vi "Read Config Unitest.vi"(8 "error in (no error)":errorcluster, 11 "main ref":T1) -> (0 "error out":errorcluster)   [LabVIEW 2025]
uses:
  controls/LAB-IQ UI Data.ctl
  Traction Loop/Traction Receipe Enum.ctl
  Config file  FGV Unitest enum.ctl
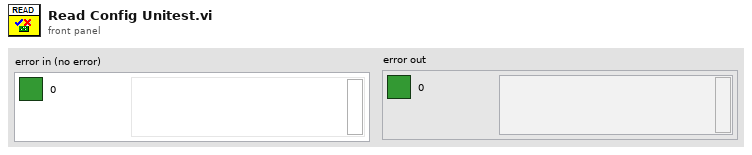
[diagram p1: front panel]
types:
  T1 = typedef "LAB-IQ UI Data.ctl" = cluster{"Main Home Screen":cluster{"GUI":refnum<vi>, "Platform Settings":refnum<vi>, "Configure":refnum<vi>, "Home":refnum<vi>, "EXIT":refnum<vi>, "service 2":refnum<vi>, "MainPage":refnum<vi>, "Analysis":refnum<vi>}, "Platform Settings":cluster{"mm/s  Surge":refnum<vi>, "Update Surge Speed":refnum<vi>, "Drive Error":refnum<vi>, "Disable Axis Jog Soft Limits":refnum<vi>, "mm/s  Sway":refnum<vi>, "Sway and Surge COM Status":refnum<vi>, "Heave COM Status":refnum<vi>, "Enable Platform":refnum<vi>, "Surge Forward Main":refnum<vi>, "Sway Right Main":refnum<vi>, "Sway Left Main":refnum<vi>, "Heave Down Main":refnum<vi>, "Heave Up main":refnum<vi>, "Update Sway Speed":refnum<vi>, "Update Heave Speed":refnum<vi>, "mm/s Heave":refnum<vi>, "mm/sec":refnum<vi>, "mm":refnum<vi>, "Surge Backward Main":refnum<vi>}, "Analysis Screen":cluster{"Analysis Home":refnum<vi>, "Surface Analysis":refnum<vi>, "Imaging":refnum<vi>, "Image Analysis":refnum<vi>, "Post Analysis":refnum<vi>}, "Config Screen":cluster{"Select Load Head":refnum<vi>, "Notes :":refnum<vi>, "FILE":refnum<vi>, "Sample ID :":refnum<vi>, "Operator ID :":refnum<vi>, "Operator Name :":refnum<vi>, "Auto":refnum<vi>}, "Motion Module":cluster{"zNL":refnum<vi>, "NL disp":refnum<vi>, "Rotary Tab":refnum<vi>, "Motion Direction:  3":refnum<vi>, "E.Velocity 2":refnum<vi>, "e.v/ssr 2":refnum<vi>, "Enter Fixed E.Velocity 2":refnum<vi>, "Enter Final SRR 2":refnum<vi>, "Enter initial SRR 2":refnum<vi>, "Enter Fixed SRR 2":refnum<vi>, "Enter the Final E.Velocity (m/s) 2":refnum<vi>, "Enter initial E.Velocity (m/s) 2":refnum<vi>, "Final Speed (RPM) 3":refnum<vi>, "Initial Speed (RPM) 2":refnum<vi>, "Enter the Final Velocity (m/s) 3":refnum<vi>, "Enter initial Velocity (m/s)  3":refnum<vi>, "Ramp Up 2":refnum<vi>, "TEST SELECTION":refnum<vi>, "SPEED SELECTION : ":refnum<vi>, "Angular Oscillation Set":refnum<vi>, "Traction":refnum<vi>, "Step Speed":refnum<vi>, "StepTable For Load-Speed":refnum<vi>, "StepTable For Speed":refnum<vi>, "Surge Forward MM":refnum<vi>, "Surge Backward MM":refnum<vi>, "M3 Image":refnum<vi>, "String 39":refnum<vi>, "Sway Left MM":refnum<vi>, "Sway Right MM":refnum<vi>, "Disable Axis Jog Soft Limits":refnum<vi>, "mm":refnum<vi>, "Heave Down MM":refnum<vi>, "Heave Up MM":refnum<vi>, "Wear Track Diameter (mm)":refnum<vi>, "Set WTD":refnum<vi>, "HomeScratch":refnum<vi>, "HomeRot":refnum<vi>, "PlaceModule":refnum<vi>, "Enter the Angle (Deg)":refnum<vi>, "Enter the Frequency (Hz)":refnum<vi>, "Motion Mode:":refnum<vi>, "LR Sway":refnum<vi>, "Rot Hor":refnum<vi>, "Scratch":refnum<vi>, "LR Cam":refnum<vi>, "MMBack":refnum<vi>, "MMNext":refnum<vi>, "Rot Ver":refnum<vi>, "Rotary Module Selection":refnum<vi>, "calculate rotary":refnum<vi>, "SPEED SELECTION : rotary":refnum<vi>, "Import 2":refnum<vi>, "Save 2":refnum<vi>, "File Path :  2":refnum<vi>, "String 45":refnum<vi>, "StepTable For Speed 3":refnum<vi>, "Enter the Speed(mm/sec)":refnum<vi>, "Enter the Speed(RPM)":refnum<vi>, "Enter Scratch Speed (mm/s):":refnum<vi>, "SwaySpeed Set":refnum<vi>, "Scartch Offset":refnum<vi>, "Motion type:":refnum<vi>, "HomeScratch 2":refnum<vi>, "Enter Scratch length (mm):":refnum<vi>, "Wear Track Diameter":refnum<vi>, "Rotary Speed Exced":refnum<vi>, "Scratch Mode":refnum<vi>, "No of Scratch":refnum<vi>}, "Environmental control":cluster{"Humidity  Status  3":refnum<vi>, "Low Temp  Status  2":refnum<vi>, "TK4 status 2":refnum<vi>, "Stage Temperature":refnum<vi>, "Sample Temperature":refnum<vi>, "Humidity (Amb)":refnum<vi>, "Clear List":refnum<vi>, "Add to list":refnum<vi>, "Wear":refnum<vi>, "Vibration":refnum<vi>, "Humidity (Chamber)":refnum<vi>, "Temperature (Chamber)":refnum<vi>, "ECR ":refnum<vi>, "Temperature (Amb)":refnum<vi>, "Microphone":refnum<vi>, "Acoustic Emission 3":refnum<vi>, "SNext":refnum<vi>, "APBack":refnum<vi>, "Enter the Temperature (°C):":refnum<vi>, "Enter the Stage \nTemperature (°C):":refnum<vi>, "Enter the Humidity (%Rh):":refnum<vi>, "Low Temp":refnum<vi>, "High Temp":refnum<vi>, "Humidity":refnum<vi>, "Sensors Picked":refnum<vi>}, "About Screen":cluster{"Password":refnum<vi>, "Home Service":refnum<vi>, "Advanced Setting":refnum<vi>, "About Tab":refnum<vi>, "ECR Port:":refnum<vi>, "Ramp Port:":refnum<vi>, "Installation/Replacement completed":refnum<vi>, "Loahead":refnum<vi>, "Heave and Surge COM Port:":refnum<vi>, "Sway COM Port:":refnum<vi>, "Temp Modbus:":refnum<vi>, "Humidity Port:":refnum<vi>, "Edit Gain Constants":refnum<vi>, "Save Gain Constants":refnum<vi>}, "Main Screen":cluster{"Main Screen Tab":refnum<vi>, "Angle and Frequency":refnum<vi>, "Stroke (mm)":refnum<vi>, "Angle (Deg)":refnum<vi>, "Main Speed Tab":refnum<vi>, "MTM MOTOR DISPLAY":refnum<vi>, "Disc Speed (m/sec)":refnum<vi>, "Ball Speed (m/sec)":refnum<vi>, "Disc Speed (RPM)":refnum<vi>, "Ball Speed (RPM)":refnum<vi>, "SPEED TAB":refnum<vi>, "Speed (m/sec)":refnum<vi>, "Set Speed (m/sec)":refnum<vi>, "Speed (RPM)":refnum<vi>, "Set Speed":refnum<vi>, "Time Tab":refnum<vi>, "Time ( HH:MM:SS ) 2":refnum<vi>, "Test Duration":refnum<vi>, "Test Duration 4":refnum<vi>, "TEST CYCLE":refnum<vi>, "TOTAL CYCLES":refnum<vi>, "Set Load (N)":refnum<vi>, "Temp Tabs":refnum<vi>, "Heater":refnum<vi>, "TK4 status":refnum<vi>, "ChamberTemp":refnum<vi>, "SetTmp":refnum<vi>, "Controller  Status":refnum<vi>, "ChamberTemp 2":refnum<vi>, "SetTmp 2":refnum<vi>, "Controller  Status 2":refnum<vi>, "ChamberTemp 3":refnum<vi>, "SetTmp 3":refnum<vi>, "Cooling":refnum<vi>, "Load Communication":refnum<vi>, "Ambient \nTemperature":refnum<vi>, "HumCOMStatus":refnum<vi>, "Ambient\n Humidity":refnum<vi>, "Freq (Hz)":refnum<vi>, "Load En":refnum<vi>, "NLt":refnum<vi>, "zNL 2":refnum<vi>, "Humidity On":refnum<vi>, "humidity disp":refnum<vi>, "Set Humidity":refnum<vi>, "NL disp 2":refnum<vi>, "Humidity On 2":refnum<vi>, "humidity disp 2":refnum<vi>, "Set Humidity 2":refnum<vi>, "NL disp 3":refnum<vi>, "AppLoadSeq scratch":refnum<vi>, "Stop Scratch":refnum<vi>, "ClrLog":refnum<vi>, "Trip Log":refnum<vi>, "STOP":refnum<vi>, "Start Test":refnum<vi>, "Test status":refnum<vi>, "AR Led":refnum<vi>, "Data":refnum<vi>, "Health":refnum<vi>, "Sway COM Status":refnum<vi>, "Heave COM Status":refnum<vi>, "Grp Tab":refnum<vi>, "Sub Graph":refnum<vi>, "SD (mm)":refnum<vi>, "Siliding distance Reset Graph":refnum<vi>, "SDGp":refnum<vi>, "Humidity Reset Graph":refnum<vi>, "HumrGp":refnum<vi>, "Acoustic Emission (mV)":refnum<vi>, "Aqucostic Reset Graph":refnum<vi>, "gACQUOS":refnum<vi>, "ECR RESET":refnum<vi>, "ECR":refnum<vi>, "Temperature Reset":refnum<vi>, "Acoustic Emission (mV) 2":refnum<vi>, "Aqucostic Reset Graph 2":refnum<vi>, "gACQUOS 2":refnum<vi>, "ECR RESET 2":refnum<vi>, "ECR 2":refnum<vi>, "Temperature Reset 2":refnum<vi>, "Temperature (deg c)":refnum<vi>, "Speed Reset Graph":refnum<vi>, "Speed Tab":refnum<vi>, "MTM DISC  SPEED":refnum<vi>, "MTM BALL SPEED":refnum<vi>, "speed mm/sec":refnum<vi>, "Hymidity":refnum<vi>, "Humidity Disable trip":refnum<vi>, "CoF Trip  2":refnum<vi>, "Depth Trip":refnum<vi>, "Weart Deapth":refnum<vi>, "Depth Reset Graph":refnum<vi>, "Weart":refnum<vi>, "Depthz":refnum<vi>, "Depth (µm)":refnum<vi>, "WearGp":refnum<vi>, "NL Trip 2":refnum<vi>, "Load pid":refnum<vi>, "Load Disable Trip":refnum<vi>, "Load Reset Graph":refnum<vi>, "NL Display 4":refnum<vi>, "Main Chart 3":refnum<vi>, "BACK":refnum<vi>, "Depth Trip 2":refnum<vi>, "COF TRIP ":refnum<vi>, "Friction Force (N)":refnum<vi>, "FF Reset Graph":refnum<vi>, "FF Disable Trip":refnum<vi>, "FF TRIP":refnum<vi>, "COF Disable Trip":refnum<vi>, "COF Reset Graph":refnum<vi>, "Start Test Temp":refnum<vi>, "zFF":refnum<vi>, "Friction Force (N) Graph":refnum<vi>, "Coefficient of Friction":refnum<vi>, "Scratch Start Test":refnum<vi>, "FF Tab":refnum<vi>, "Cyclic Friction Force (N)":refnum<vi>, "CZ FF":refnum<vi>, "Cyclic Friction Force (N) Graph":refnum<vi>, "Cyclic Coefficient of Friction":refnum<vi>, "Cyclic FF TRIP":refnum<vi>, "Cyclic FF Disable Trip":refnum<vi>, "cyclic COF Disable Trip":refnum<vi>, "cyclic COF TRIP":refnum<vi>, "cyclic COF Reset Graph":refnum<vi>, "Cyclic FF Reset Graph":refnum<vi>, "Test Trip":refnum<vi>, "Multi Scratch Pass":refnum<vi>, "Scratch Start Recording":refnum<vi>}, "Loading":cluster{"Indentation":refnum<vi>, "Reference Sample":refnum<vi>, "Load Cell Communication Slide":refnum<vi>, "com 3":refnum<vi>, "com":refnum<vi>, "DecaForce COM Status":refnum<vi>, "Update":refnum<vi>, "Clear 3":refnum<vi>, "seq":refnum<vi>, "Stribeck table":refnum<vi>, "Stribeck Table  For loading":refnum<vi>, "Loading Mode":refnum<vi>, "Enter the Final Load (N)":refnum<vi>, "Enter the CoF Trip":refnum<vi>, "Enter the Friction Force Trip":refnum<vi>, "Enter the Normal load Trip":refnum<vi>, "Enter the Load  (N)":refnum<vi>, "KiloForce":refnum<vi>, "DecaForce ":refnum<vi>, "MicroForce":refnum<vi>, "LHBack":refnum<vi>, "LHNext":refnum<vi>, "Enter the Loading Rate (N/min)":refnum<vi>, "Message":refnum<vi>, "Warning 2":refnum<vi>, "SSP 0.75":refnum<vi>, "SSP 0.5":refnum<vi>, "SSP 0.3":refnum<vi>, "Warning":refnum<vi>, "gui GIF":refnum<vi>, "Communication is established":refnum<vi>, "AppLoad 4":refnum<vi>, "Multipoint":refnum<vi>, "Load Selection":refnum<vi>}, "PID":cluster{"Ramp MulFac":refnum<vi>, "pulses LoadDiffRamp(2..10)":refnum<vi>, "PulseControlRamp(diff<=3N)":refnum<vi>, "SetLoadDeadband(%) Load(0-10N)":refnum<vi>, "PID gains out delay (microForce)":refnum<vi>, "Ramp":refnum<vi>, "Gain 2":refnum<vi>, "pulses LoadDiff(2..10)":refnum<vi>, "pulses LoadDiff(11..50)":refnum<vi>, "PulseControl(diff<=3N)":refnum<vi>, "SetLoadDeadband(%)  2":refnum<vi>, "Dummy Run":refnum<vi>, "Vertical load (N)":refnum<vi>, "AutoTune":refnum<vi>, "Offset 3 ":refnum<vi>, "apply load":refnum<vi>, "Offset  3":refnum<vi>, "apply load 2":refnum<vi>, "Enter ByPass Load":refnum<vi>, "reinit 3":refnum<vi>, "output range delay":refnum<vi>, "PID gains out delay":refnum<vi>, "Bypass Load":refnum<vi>, "pulsesSent":refnum<vi>, "pulses ":refnum<vi>, "actpid":refnum<vi>, "gFF Rot":refnum<vi>, "pulses LoadDiff(21..1000)":refnum<vi>, "Delay":refnum<vi>, "deadband":refnum<vi>}, "Config Parameters":cluster{"Tab Control 3":refnum<vi>, "Tab Control 19":refnum<vi>, "SAMPLES":refnum<vi>, "Re-initilaize":refnum<vi>, "Filter ON/OFF":refnum<vi>, "TracHomeSurgeOffsetCounts 10MM":refnum<vi>, "TracHomeSwayOffsetCounts 10MM":refnum<vi>, "Acoustic Emission:":refnum<vi>, "Apply Filter (FF)":refnum<vi>, "Filter% 2":refnum<vi>, "Apply Filter (Load)":refnum<vi>, "Filter% ":refnum<vi>, "Sway distance (mm)":refnum<vi>, "Surge distance (mm)":refnum<vi>, "DataSavingLoopDelay(ms)":refnum<vi>, "SAVE 2":refnum<vi>, "Enter Distance":refnum<vi>, "Sway Counts:":refnum<vi>, "Distance (mm): 3":refnum<vi>, "Surge Counts:":refnum<vi>, "Distance (mm): 2":refnum<vi>, "Distance (mm):":refnum<vi>, "Heave Counts:":refnum<vi>, "LRMHomeSurgeOffsetCounts":refnum<vi>, "LRMHomeSwayOffsetCounts":refnum<vi>, "TracHomeSurgeOffsetCounts 20MM":refnum<vi>, "TracHomeSwayOffsetCounts 20MM":refnum<vi>, "RotHomeSwayOffsetCounts":refnum<vi>, "RotHomeSurgeOffsetCounts":refnum<vi>, "Heave distance":refnum<vi>, "Zmm":refnum<vi>, "Heave Pulses/mm":refnum<vi>, "Surge Pulses/mm":refnum<vi>, "Sway Pulses/mm":refnum<vi>, "Heave Pitch":refnum<vi>, "Surge Pitch":refnum<vi>, "Sway Pitch":refnum<vi>, "Heave PPR":refnum<vi>, "Surge PPR":refnum<vi>, "Sway PPR":refnum<vi>, "Tab Control 5":refnum<vi>, "Tab Control 14":refnum<vi>, "Tab Control 26":refnum<vi>, "AE":refnum<vi>, "Heave Loop Delay":refnum<vi>, "Heave PID Speed":refnum<vi>, "Surge Jog Speed":refnum<vi>, "Heave Jog Speed":refnum<vi>, "Sway Loop Delay":refnum<vi>, "Sway PID Speed":refnum<vi>, "Sway Jog Speed":refnum<vi>, "DEPTH TRIP VALUE":refnum<vi>, "LOAD TRIP VALUE":refnum<vi>, "DEPTH TRIP   ENABLE":refnum<vi>, "LOAD TRIP  ENABLE":refnum<vi>, "CYCLIC FF TRIP VALUE":refnum<vi>, "FF TRIP VALUE":refnum<vi>, "CYCLIC CoF TRIP VALUE":refnum<vi>, "COF TRIP VALUE":refnum<vi>, "CYCLIC COF TRIP  ENABLE":refnum<vi>, "CYCLIC FF TRIP  ENABLE":refnum<vi>, "FF TRIP  ENABLE":refnum<vi>, "COF TRIP  ENABLE":refnum<vi>, "JOG TRIP LOAD VALUE (N)":refnum<vi>, "Rotary Vertical":refnum<vi>, "Traction":refnum<vi>, "Scratch":refnum<vi>, "LRM CAM":refnum<vi>, "Sway LRM":refnum<vi>, "Rotary Horizontal":refnum<vi>}, "Loading Com Port":cluster{"ClearAll":refnum<vi>, "Mz(Nm)":refnum<vi>, "My(Nm)":refnum<vi>, "Mx(Nm)":refnum<vi>, "Save Dwell":refnum<vi>, "Acq Delay (ms)":refnum<vi>, "Burst Delay (ms)":refnum<vi>, "model":refnum<vi>, "SN":refnum<vi>, "FFx(N)":refnum<vi>, "Sensor IP":refnum<vi>, "Port":refnum<vi>, "FFy(N)":refnum<vi>, "Load(N)":refnum<vi>, "delete Handle":refnum<vi>, "Create Handle":refnum<vi>, "ft_data":refnum<vi>, "ft_range":refnum<vi>, "ft_data 2":refnum<vi>, "stop 6":refnum<vi>, "running_flag":refnum<vi>, "ft_udp_handle":refnum<vi>, "get-data-return":refnum<vi>, "get-range-return":refnum<vi>, "zero-return":refnum<vi>, "filter-return":refnum<vi>, "initial-return":refnum<vi>, "deleteHandle-result":refnum<vi>, "Load Cell Temp":refnum<vi>, "Load Cell":refnum<vi>, "ZeroAll":refnum<vi>, "FORCE (N)":refnum<vi>, "TORQUE (N-m)":refnum<vi>}, "Heave AND Surge":cluster{"SURGE POSE":refnum<vi>, "error out Read":refnum<vi>, "HEAVE POSE":refnum<vi>, "State":refnum<vi>, "Homed":refnum<vi>, "Sequence ID":refnum<vi>, "error out Write":refnum<vi>, "faultCode":refnum<vi>, "Ack ID":refnum<vi>, "SPEED":refnum<vi>, "Distance":refnum<vi>, "Mode Command":refnum<vi>, "Heave and Surge Read":refnum<vi>, "Read Heave Temp":refnum<vi>, "Spare 15":refnum<vi>, "Spare 14":refnum<vi>, "Spare 13":refnum<vi>, "Spare 12":refnum<vi>, "Spare 11":refnum<vi>, "Spare 10":refnum<vi>, "Spare 9":refnum<vi>, "Spare 8":refnum<vi>, "Spare 7":refnum<vi>, "Spare 6":refnum<vi>, "Spare 5":refnum<vi>, "Spare 4":refnum<vi>, "Spare 2":refnum<vi>, "Spare 1":refnum<vi>, "Node Id":refnum<vi>, "Spare 3":refnum<vi>, "SPARE 4":refnum<vi>, "SPARE 3":refnum<vi>, "SPARE 2":refnum<vi>, "SPARE 1":refnum<vi>, "fwMajor":refnum<vi>, "fwMinor":refnum<vi>, "Manual Write":refnum<vi>, "Heave and Surge Write":refnum<vi>, "SPARE 5":refnum<vi>, "Reserved ":refnum<vi>, "SPARE 8":refnum<vi>, "SPARE 6":refnum<vi>, "SPARE 7":refnum<vi>, "SPARE 17":refnum<vi>, "SPARE 16":refnum<vi>, "SPARE 15":refnum<vi>, "SPARE 14":refnum<vi>, "SPARE 13":refnum<vi>, "SPARE 12":refnum<vi>, "SPARE 11":refnum<vi>, "SPARE 10":refnum<vi>, "SPARE 9":refnum<vi>, "System UPTIME":refnum<vi>, "Missed Packets":refnum<vi>, "faultCode Surge Right":refnum<vi>, "faultCode Surge Left":refnum<vi>, "faultCode Heave":refnum<vi>, "UPLINK HEAVE":refnum<vi>, "DOWNLINK HEAVE":refnum<vi>}, "New PID LOGIC":cluster{"Fine Tune Zone":refnum<vi>, "PID SDelay":refnum<vi>, "Max_pos_limit":refnum<vi>, "Min_pos_limit":refnum<vi>, "i_limit":refnum<vi>, "pct_scale":refnum<vi>, "Deadband":refnum<vi>, "Kd":refnum<vi>, "Ki":refnum<vi>, "Kp":refnum<vi>, "Current Position":refnum<vi>, "Set Load":refnum<vi>, "Current Load":refnum<vi>, "Pulse delta":refnum<vi>, "Init Step":refnum<vi>, "Max Step Linit":refnum<vi>, "min_deadband_floor":refnum<vi>, "dynamic_spindle_noise_scalar":refnum<vi>, "min_finetune_floor":refnum<vi>, "filter_alpha":refnum<vi>, "PID":refnum<vi>}, "SWAY ":cluster{"fwMajor":refnum<vi>, "Homed":refnum<vi>, "Rotary POSE":refnum<vi>, "State":refnum<vi>, "SWAY POSE":refnum<vi>, "Ack ID":refnum<vi>, "faultCode":refnum<vi>, "Node Id":refnum<vi>, "fwMinor":refnum<vi>, "Spare 6":refnum<vi>, "Spare 5":refnum<vi>, "Spare 4":refnum<vi>, "Spare 3":refnum<vi>, "Spare 2":refnum<vi>, "Spare 1":refnum<vi>, "Spare 7":refnum<vi>, "SPARE  5":refnum<vi>, "error out Write  SWAY ":refnum<vi>, "error out Read SWAY ":refnum<vi>, "Manual Write SWAY ":refnum<vi>, "SWAY WRITE":refnum<vi>, "SPARE  4":refnum<vi>, "SPARE  3":refnum<vi>, "SPARE 2":refnum<vi>, "SPARE 1":refnum<vi>, "Spare 15":refnum<vi>, "Spare 14":refnum<vi>, "Spare 13":refnum<vi>, "Spare 12":refnum<vi>, "Spare 11":refnum<vi>, "Spare 9":refnum<vi>, "Spare 8":refnum<vi>, "SPEED":refnum<vi>, "Distance":refnum<vi>, "Mode Command":refnum<vi>, "Sequence ID":refnum<vi>, "SWAY READ":refnum<vi>, "Spare 10":refnum<vi>, "Read SWAY Temp":refnum<vi>, "faultCode Sway ":refnum<vi>, "Missed Packets":refnum<vi>, "System UPTIME sway":refnum<vi>, "SPARE 6":refnum<vi>, "SPARE 7":refnum<vi>, "SPARE 9":refnum<vi>, "SPARE 11":refnum<vi>, "SPARE 10":refnum<vi>, "SPARE 8":refnum<vi>, "SPARE 13":refnum<vi>, "SPARE 12":refnum<vi>, "SPARE 17":refnum<vi>, "SPARE 16":refnum<vi>, "SPARE 15":refnum<vi>, "SPARE 14":refnum<vi>, "Reserved":refnum<vi>, "faultCode Rotary":refnum<vi>, "UPLINK SWAY":refnum<vi>, "DOWNLINK SWAY":refnum<vi>}, "Analysis Screen":cluster{"Analysis Home":refnum<vi>, "Refresh 2":refnum<vi>, "MEAN 4":refnum<vi>, "SD 4":refnum<vi>, "VARIANCE 4":refnum<vi>, "MEAN  3":refnum<vi>, "SD  3":refnum<vi>, "VARIANCE  3":refnum<vi>, "MEAN 2":refnum<vi>, "SD  2":refnum<vi>, "VARIANCE 2":refnum<vi>, "MEAN":refnum<vi>, "SD":refnum<vi>, "VARIANCE":refnum<vi>, "File 4 Discription":refnum<vi>, "OPEN 4":refnum<vi>, "File Name 4":refnum<vi>, "OPEN 3":refnum<vi>, "File 3 Discription":refnum<vi>, "File Name 3":refnum<vi>, "Y-AXIS":refnum<vi>, "X-AXIS":refnum<vi>, "XY Graph":refnum<vi>, "File Name 2":refnum<vi>, "File Name 1":refnum<vi>, "OPEN 2":refnum<vi>, "OPEN 1":refnum<vi>, "File 1 Discription ":refnum<vi>, "File 2 Discription":refnum<vi>, "Export":refnum<vi>, "File Format":refnum<vi>}, "Traction":cluster{"faultCode Traction 2":refnum<vi>, "faultCode Traction 1":refnum<vi>, "Missed Packets":refnum<vi>, "System UPTIME Traction":refnum<vi>, "SPARE 17":refnum<vi>, "SPARE 16":refnum<vi>, "SPARE 15":refnum<vi>, "SPARE 14":refnum<vi>, "SPARE 13":refnum<vi>, "SPARE 12":refnum<vi>, "SPARE 11":refnum<vi>, "SPARE 10":refnum<vi>, "SPARE 9":refnum<vi>, "SPARE 8":refnum<vi>, "SPARE 7":refnum<vi>, "SPARE 6":refnum<vi>, "Reserved":refnum<vi>, "SPARE  5":refnum<vi>, "Manual Write TRACTION":refnum<vi>, "TRACTION WRITE":refnum<vi>, "SPARE  4":refnum<vi>, "SPARE  3":refnum<vi>, "SPARE 2":refnum<vi>, "SPARE 1":refnum<vi>, "Spare 7":refnum<vi>, "Spare 6":refnum<vi>, "Spare 5":refnum<vi>, "Spare 4":refnum<vi>, "Spare 2":refnum<vi>, "Spare 1":refnum<vi>, "Node Id":refnum<vi>, "Read TRACTION Temp":refnum<vi>, "fwMinor":refnum<vi>, "fwMajor":refnum<vi>, "faultCode":refnum<vi>, "TRACTION POSE":refnum<vi>, "TRACTION POSE 2":refnum<vi>, "Homed":refnum<vi>, "State":refnum<vi>, "Ack ID":refnum<vi>, "SPEED":refnum<vi>, "Distance":refnum<vi>, "Mode Command":refnum<vi>, "Sequence ID":refnum<vi>, "error out Read TRACTION":refnum<vi>, "error out Write  TRACTION":refnum<vi>, "TRACTION READ":refnum<vi>, "Spare 3":refnum<vi>, "Downlink traction":refnum<vi>, "Uplink Traction":refnum<vi>}, "Traction reciepe":cluster{"SRR Sweep Range (%) Stribeck":refnum<vi>, "Traction Receipe":refnum<vi>, "Total Execution Time":refnum<vi>, "Total Steps":refnum<vi>, "Duration / Step (s)  Stribeck":refnum<vi>, "STRIBECK Fixed SRR List (%)":refnum<vi>, "Duration / Step (s) Traction":refnum<vi>, "SRR Sweep Range (%) traction":refnum<vi>, "Rolling Speed (mm/s)":refnum<vi>, "Temperature Stages (°C)":refnum<vi>, "Ball Load (N)":refnum<vi>, "Lubricant Name":refnum<vi>, "Profile File Name":refnum<vi>, "SET entrainment Velocity":refnum<vi>, "Test Array Size":refnum<vi>, "SRR INDEX [ STRIBECK]":refnum<vi>, "Stribeck Size":refnum<vi>, "SET SRR":refnum<vi>, "ELAPSED TIMER ":refnum<vi>, "BALL SET RPM":refnum<vi>, "DISC SET RPM":refnum<vi>, "SET LOAD":refnum<vi>, "TEMPERATURE READ":refnum<vi>, "SET TEMPERATURE":refnum<vi>, "Traction Size":refnum<vi>, "DISC SPEED (rpm)":refnum<vi>, "BALL SPEED (rpm)":refnum<vi>, "BALL WEAR TRACK":refnum<vi>, "DISC WEARTRACK":refnum<vi>, "SRR INDEX [ TRACTION]":refnum<vi>, "Start Index Type":refnum<vi>, "Enum - Menu":refnum<vi>, "Ball (mm/sec)":refnum<vi>, "Disc (mm/sec)":refnum<vi>}, "Traction Control":cluster{"HomeTraction":refnum<vi>, "Demo Mode Display":refnum<vi>, "Traction Message":refnum<vi>, "Traction Step Update Details":refnum<vi>, "Main Tab sequence for selection":refnum<vi>, "Ramp Tab":refnum<vi>, "e.v/ssr":refnum<vi>, "Enter Fixed E.Velocity":refnum<vi>, "Enter Final SRR":refnum<vi>, "Enter initial SRR":refnum<vi>, "Enter Fixed SRR":refnum<vi>, "Enter the Final E.Velocity (m/s)":refnum<vi>, "Enter initial E.Velocity (m/s)":refnum<vi>, "Ball WTD":refnum<vi>, "E.Velocity":refnum<vi>, "Enter the Final Velocity (m/s)":refnum<vi>, "Enter initial Velocity (m/s)":refnum<vi>, "Ramp Up   Disc":refnum<vi>, "Initial DiscSpeed (RPM)":refnum<vi>, "Final Speed (RPM) Ball":refnum<vi>, "Final Speed (RPM)":refnum<vi>, "Initial Speed (RPM) Ball":refnum<vi>, "Enter the Final Velocity (m/s) Ball":refnum<vi>, "Enter initial Velocity (m/s) Ball":refnum<vi>, "Ramp Up":refnum<vi>, "ExceedBallSpeed step":refnum<vi>, "ExceedDiscSpeed":refnum<vi>, "BallSpeed Exceed Indication":refnum<vi>, "Apply":refnum<vi>, "SPEED SELECTION : MTM":refnum<vi>, "SPEED SELECTION : MTM 2":refnum<vi>, "TEST SELECTION (MTM)":refnum<vi>, "MTM Test Selection":refnum<vi>, "File Path Tab":refnum<vi>, "File Path String":refnum<vi>, "Save":refnum<vi>, "Save  2":refnum<vi>, "Import ":refnum<vi>, "File Path :":refnum<vi>, "Step Sequence Indication Tab":refnum<vi>, "Step Sequence Indication":refnum<vi>, "Calculate Step":refnum<vi>, "StepTable":refnum<vi>, "ExceedDiscSpeed  Cinstant Speed":refnum<vi>, "ExceedBallSpeed Constant":refnum<vi>, "TEST SELECTION (MTM) 2":refnum<vi>, "SPEED SELECTION : MTM 3":refnum<vi>, "MTM Test Selection 2":refnum<vi>, "Enter the Speed (m/sec): ":refnum<vi>, "Enter the Speed (m/sec):  2":refnum<vi>, "Enter the Speed (RPM):":refnum<vi>, "Lower Spped ":refnum<vi>, "Upper":refnum<vi>, "Enter the Speed (RPM):Ball":refnum<vi>, "Disc Motion Direction: ":refnum<vi>, "Ball Motion Direction :":refnum<vi>, "Motion Mode: ":refnum<vi>, "Wear Track Diameter (mm) ":refnum<vi>, "Disc Speed Indicator":refnum<vi>, "ExceedBallSpeed":refnum<vi>}, "Acquostic":cluster{"Last Config Rejected ":refnum<vi>, "rx command count":refnum<vi>, "Current Filter Id":refnum<vi>, "Isolated Gain":refnum<vi>, "DAQ Status":refnum<vi>, "error out":refnum<vi>, "error in (no error)":refnum<vi>, "Uplink Packet":refnum<vi>, "data out":refnum<vi>, "Downlink Packet":refnum<vi>, "Signal Energy":refnum<vi>, "Amplitude db_AE":refnum<vi>, "Peak Amplitude":refnum<vi>, "AE Ring-Down Counts":refnum<vi>, "Gains":refnum<vi>, "Manual Write Acquostic":refnum<vi>}}
  T2 = typedef "Config file  FGV Unitest enum.ctl" = enum16{"OPEN", "READ", "WRITE", "CLOSE"}
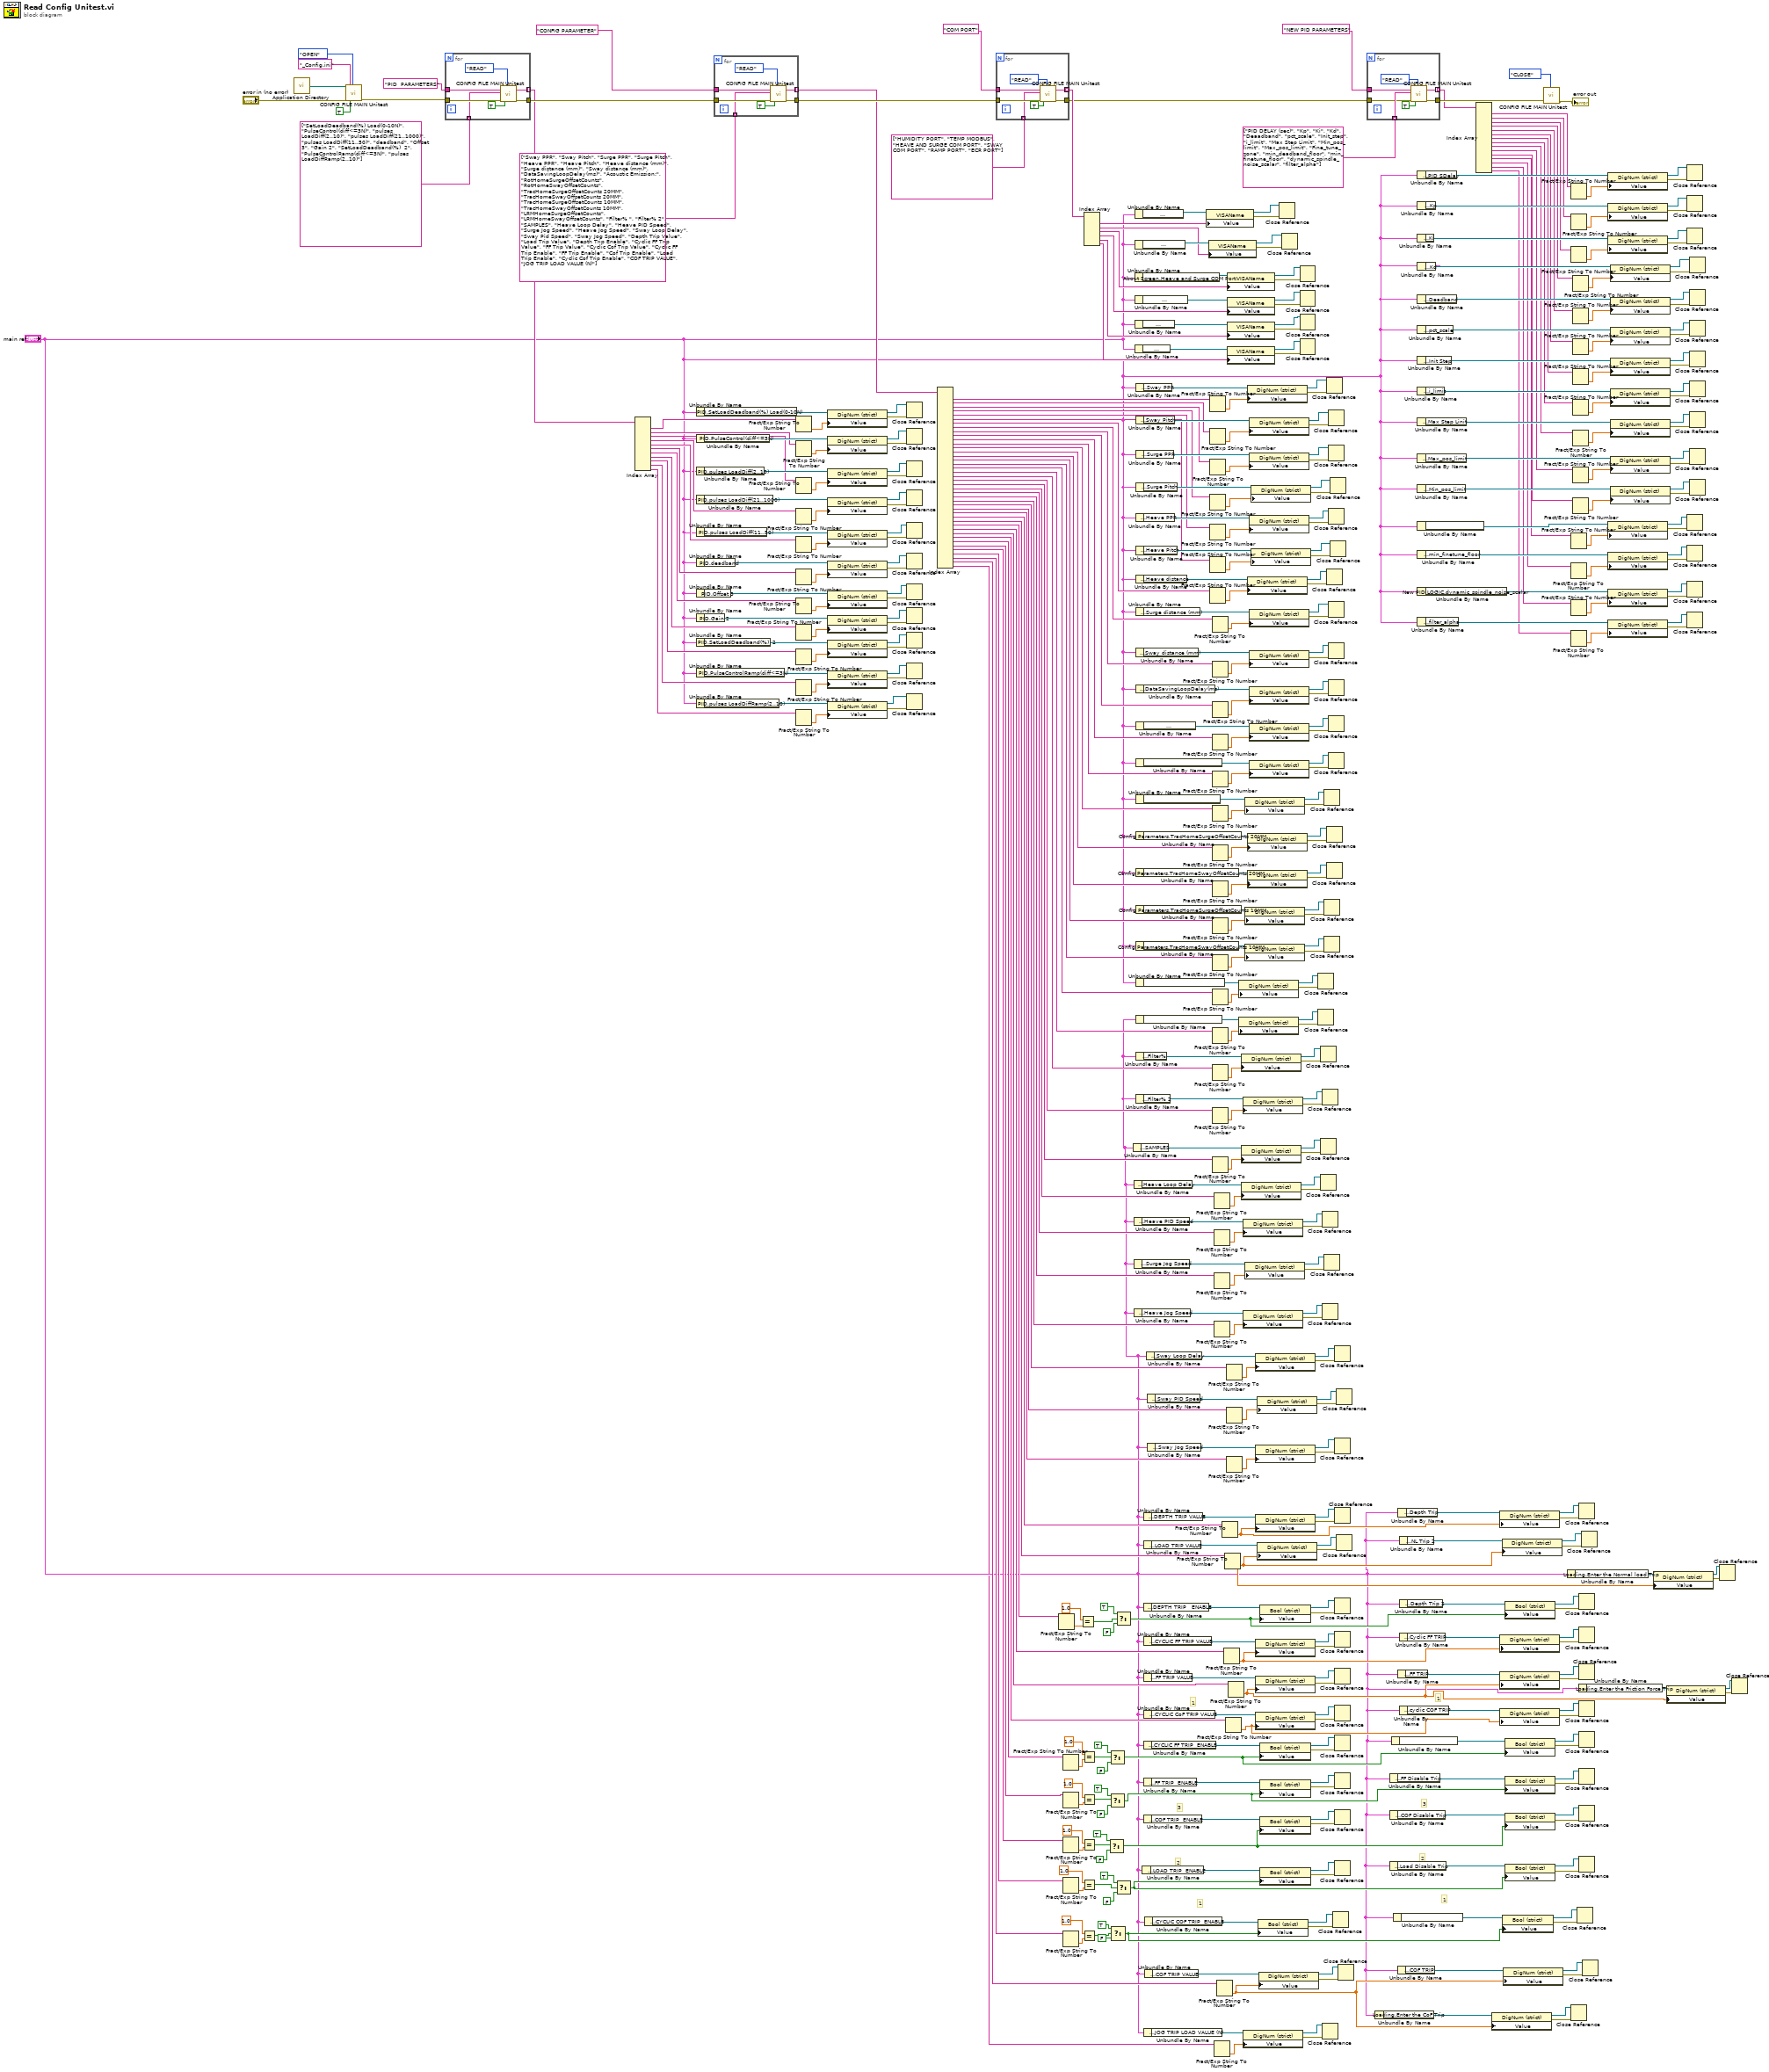
[diagram p0: block diagram]
diagram:
  # "3"
  # "2"
  # "1"
  # "1"
  # "3"
  # "2"
  # "1"
  # "1"
  n1 = call <vilib>:"Application Directory.vi"() -> ("Application Directory"=w460:path)
  n2 = call "CONFIG FILE MAIN Unitest.vi"("File Path"=w460, "error in"="error in (no error)", "file name"="_Config.ini", "PARAMETER/CONFIG"=TRUE, "Config Enum"=Config_file__FGV_Unitest_enum."OPEN") -> ("error out"=w459:errorcluster)  [unwired: 13 in, 1 out]
  n3 = for {
    tunnel: w459 -> [w471]
    tunnel: "PID  PARAMETERS" ("WRITE /READ SECTION") -> [w470]
    tunnel: string[] ["SetLoadDeadband(%) Load(0-10N)", "PulseControl(diff<=3N)", "pulses LoadDiff(2..10)", "pulses LoadDiff(21..1000)", "pulses LoadDiff(11..50)", "deadband", "Offset  3", "Gain 2", "SetLoadDeadband(%)  2", "PulseControlRamp(diff<=3N)", "pulses LoadDiffRamp(2..10)"] -> [w466] mode=indexing
    tunnel: [w469] -> w456
    tunnel: [w465] -> w269 mode=indexing
    n4 = call "CONFIG FILE MAIN Unitest.vi"("WRITE /READ SECTION"=w470, "READ KEY"=w466, "error in"=w471, "PARAMETER/CONFIG"=TRUE, "Config Enum"=Config_file__FGV_Unitest_enum."READ") -> ("READ VALUE"=w465:string, "error out"=w469:errorcluster)  [unwired: 13 in]
  }
  n5 = Index Array(array=w269) -> (element #1=w268:string, element #2=w267:string, element #3=w266:string, element #4=w265:string, element #5=w264:string, element #6=w263:string, element #7=w262:string, element #8=w261:string, element #9=w260:string, element #10=w259:string, element #11=w258:string)  [unwired: 11 in]
  n6 = Unbundle By Name("main ref") -> ("PID.SetLoadDeadband(%) Load(0-10N)"=w450:refnum<vi>)
  n7 = Unbundle By Name("main ref") -> ("PID.PulseControl(diff<=3N)"=w445:refnum<vi>)
  n8 = Unbundle By Name("main ref") -> ("PID.pulses LoadDiff(2..10)"=w444:refnum<vi>)
  n9 = Unbundle By Name("main ref") -> ("PID.pulses LoadDiff(21..1000)"=w439:refnum<vi>)
  n10 = Unbundle By Name("main ref") -> ("PID.pulses LoadDiff(11..50)"=w438:refnum<vi>)
  n11 = Unbundle By Name("main ref") -> ("PID.deadband"=w433:refnum<vi>)
  n12 = Unbundle By Name("main ref") -> ("PID.Offset 3"=w432:refnum<vi>)
  n13 = Unbundle By Name("main ref") -> ("PID.Gain 2"=w427:refnum<vi>)
  n14 = Unbundle By Name("main ref") -> ("PID.SetLoadDeadband(%)  2"=w426:refnum<vi>)
  n15 = Unbundle By Name("main ref") -> ("PID.PulseControlRamp(diff<=3N)"=w422:refnum<vi>)
  n16 = Unbundle By Name("main ref") -> ("PID.pulses LoadDiffRamp(2..10)"=w420:refnum<vi>)
  n17 = for {
    tunnel: w456 -> [w478]
    tunnel: "CONFIG PARAMETER" ("WRITE /READ SECTION") -> [w477]
    tunnel: [w476] -> w454
    tunnel: string[] ["Sway PPR", "Sway Pitch", "Surge PPR", "Surge Pitch", "Heave PPR", "Heave Pitch", "Heave distance (mm)", "Surge distance (mm)", "Sway distance (mm)", "DataSavingLoopDelay(ms)", "Acoustic Emission:", "RotHomeSurgeOffsetCounts", "RotHomeSwayOffsetCounts", "TracHomeSurgeOffsetCounts 20MM", "TracHomeSwayOffsetCounts 20MM", "TracHomeSurgeOffsetCounts 10MM", "TracHomeSwayOffsetCounts 10MM", "LRMHomeSurgeOffsetCounts", "LRMHomeSwayOffsetCounts", "Filter% ", "Filter% 2", "SAMPLES", "Heave Loop Delay", "Heave PID Speed", "Surge Jog Speed", "Heave Jog Speed", "Sway Loop Delay", "Sway Pid Speed", "Sway Jog Speed", "Depth Trip Value", "Load Trip Value", "Depth Trip Enable", "Cyclic FF Trip Value", "FF Trip Value", "Cyclic Cof Trip Value", "Cyclic FF Trip Enable", "FF Trip Enable", "Cof Trip Enable", "Load Trip Enable", "Cyclic Cof Trip Enable", "COF TRIP VALUE", "JOG TRIP LOAD VALUE (N)"] -> [w473] mode=indexing
    tunnel: [w472] -> w325 mode=indexing
    n18 = call "CONFIG FILE MAIN Unitest.vi"("WRITE /READ SECTION"=w477, "READ KEY"=w473, "error in"=w478, "PARAMETER/CONFIG"=TRUE, "Config Enum"=Config_file__FGV_Unitest_enum."READ") -> ("READ VALUE"=w472:string, "error out"=w476:errorcluster)  [unwired: 13 in]
  }
  n19 = Fract/Exp String To Number(string=w268) -> (number=w280:dbl)  [unwired: 3 in, 1 out]
  n20 = Fract/Exp String To Number(string=w267) -> (number=w279:dbl)  [unwired: 3 in, 1 out]
  n21 = Fract/Exp String To Number(string=w266) -> (number=w278:dbl)  [unwired: 3 in, 1 out]
  n22 = Fract/Exp String To Number(string=w265) -> (number=w277:dbl)  [unwired: 3 in, 1 out]
  n23 = Fract/Exp String To Number(string=w264) -> (number=w276:dbl)  [unwired: 3 in, 1 out]
  n24 = Fract/Exp String To Number(string=w263) -> (number=w275:dbl)  [unwired: 3 in, 1 out]
  n25 = Fract/Exp String To Number(string=w262) -> (number=w274:dbl)  [unwired: 3 in, 1 out]
  n26 = Fract/Exp String To Number(string=w261) -> (number=w273:dbl)  [unwired: 3 in, 1 out]
  n27 = Fract/Exp String To Number(string=w260) -> (number=w272:dbl)  [unwired: 3 in, 1 out]
  n28 = Fract/Exp String To Number(string=w259) -> (number=w271:dbl)  [unwired: 3 in, 1 out]
  n29 = Fract/Exp String To Number(string=w258) -> (number=w270:dbl)  [unwired: 3 in, 1 out]
  n30 = property class="DigNum (strict)"(reference=w450, "Value"=w280) -> (reference out=w448:refnum<vi>, error out=w449:errorcluster)  [unwired: 1 in]
  n31 = property class="DigNum (strict)"(reference=w445, "Value"=w279) -> (reference out=w447:refnum<vi>, error out=w446:errorcluster)  [unwired: 1 in]
  n32 = property class="DigNum (strict)"(reference=w444, "Value"=w278) -> (reference out=w442:refnum<vi>, error out=w443:errorcluster)  [unwired: 1 in]
  n33 = property class="DigNum (strict)"(reference=w439, "Value"=w277) -> (reference out=w441:refnum<vi>, error out=w440:errorcluster)  [unwired: 1 in]
  n34 = property class="DigNum (strict)"(reference=w438, "Value"=w276) -> (reference out=w436:refnum<vi>, error out=w437:errorcluster)  [unwired: 1 in]
  n35 = property class="DigNum (strict)"(reference=w433, "Value"=w275) -> (reference out=w435:refnum<vi>, error out=w434:errorcluster)  [unwired: 1 in]
  n36 = property class="DigNum (strict)"(reference=w432, "Value"=w274) -> (reference out=w430:refnum<vi>, error out=w431:errorcluster)  [unwired: 1 in]
  n37 = property class="DigNum (strict)"(reference=w427, "Value"=w273) -> (reference out=w429:refnum<vi>, error out=w428:errorcluster)  [unwired: 1 in]
  n38 = property class="DigNum (strict)"(reference=w426, "Value"=w272) -> (reference out=w424:refnum<vi>, error out=w425:errorcluster)  [unwired: 1 in]
  n39 = property class="DigNum (strict)"(reference=w422, "Value"=w271) -> (reference out=w421:refnum<vi>, error out=w423:errorcluster)  [unwired: 1 in]
  n40 = property class="DigNum (strict)"(reference=w420, "Value"=w270) -> (reference out=w418:refnum<vi>, error out=w419:errorcluster)  [unwired: 1 in]
  n41 = Close Reference(reference=w448, error in (no error)=w449) -> ()  [unwired: 1 out]
  n42 = Close Reference(reference=w447, error in (no error)=w446) -> ()  [unwired: 1 out]
  n43 = Close Reference(reference=w442, error in (no error)=w443) -> ()  [unwired: 1 out]
  n44 = Close Reference(reference=w441, error in (no error)=w440) -> ()  [unwired: 1 out]
  n45 = Close Reference(reference=w436, error in (no error)=w437) -> ()  [unwired: 1 out]
  n46 = Close Reference(reference=w435, error in (no error)=w434) -> ()  [unwired: 1 out]
  n47 = Close Reference(reference=w430, error in (no error)=w431) -> ()  [unwired: 1 out]
  n48 = Close Reference(reference=w429, error in (no error)=w428) -> ()  [unwired: 1 out]
  n49 = Close Reference(reference=w424, error in (no error)=w425) -> ()  [unwired: 1 out]
  n50 = Close Reference(reference=w421, error in (no error)=w423) -> ()  [unwired: 1 out]
  n51 = Close Reference(reference=w418, error in (no error)=w419) -> ()  [unwired: 1 out]
  n52 = Index Array(array=w325) -> (element #1=w324:string, element #2=w323:string, element #3=w322:string, element #4=w321:string, element #5=w320:string, element #6=w319:string, element #7=w318:string, element #8=w317:string, element #9=w316:string, element #10=w315:string, element #11=w314:string, element #12=w313:string, element #13=w312:string, element #14=w311:string, element #15=w310:string, element #16=w309:string, element #17=w308:string, element #18=w307:string, element #19=w306:string, element #20=w305:string, element #21=w304:string, element #22=w303:string, element #23=w241:string, element #24=w240:string, element #25=w239:string, element #26=w238:string, element #27=w166:string, element #28=w165:string, element #29=w164:string, element #30=w114:string, element #31=w113:string, element #32=w112:string, element #33=w111:string, element #34=w110:string, element #35=w109:string, element #36=w108:string, element #37=w107:string, element #38=w106:string, element #39=w105:string, element #40=w104:string, element #41=w50:string, element #42=w2:string)  [unwired: 42 in]
  n53 = for {
    tunnel: w454 -> [w485]
    tunnel: "COM PORT" ("WRITE /READ SECTION") -> [w484]
    tunnel: [w483] -> w236
    tunnel: string[] ["HUMIDITY PORT", "TEMP MODBUS", "HEAVE AND SURGE COM PORT", "SWAY COM PORT", "RAMP PORT", "ECR PORT"] -> [w480] mode=indexing
    tunnel: [w479] -> w332 mode=indexing
    n54 = call "CONFIG FILE MAIN Unitest.vi"("WRITE /READ SECTION"=w484, "READ KEY"=w480, "error in"=w485, "PARAMETER/CONFIG"=TRUE, "Config Enum"=Config_file__FGV_Unitest_enum."READ") -> ("READ VALUE"=w479:string, "error out"=w483:errorcluster)  [unwired: 13 in]
  }
  n55 = Fract/Exp String To Number(string=w112) -> (number=w126:dbl)  [unwired: 3 in, 1 out]
  n56 = Fract/Exp String To Number(string=w108) -> (number=w127:dbl)  [unwired: 3 in, 1 out]
  n57 = Fract/Exp String To Number(string=w107) -> (number=w125:dbl)  [unwired: 3 in, 1 out]
  n58 = Fract/Exp String To Number(string=w106) -> (number=w124:dbl)  [unwired: 3 in, 1 out]
  n59 = Fract/Exp String To Number(string=w105) -> (number=w123:dbl)  [unwired: 3 in, 1 out]
  n60 = Fract/Exp String To Number(string=w104) -> (number=w122:dbl)  [unwired: 3 in, 1 out]
  n61 = Equal?(x=1.0, y=w126) -> (x = y?=w87:bool)
  n62 = Equal?(x=1.0, y=w127) -> (x = y?=w90:bool)
  n63 = Equal?(x=1.0, y=w125) -> (x = y?=w91:bool)
  n64 = Equal?(x=1.0, y=w124) -> (x = y?=w92:bool)
  n65 = Equal?(x=1.0, y=w123) -> (x = y?=w93:bool)
  n66 = Equal?(x=1.0, y=w122) -> (x = y?=w115:bool)
  n67 = Index Array(array=w332) -> (element #1=w331:string, element #2=w330:string, element #3=w329:string, element #4=w328:string, element #5=w327:string, element #6=w326:string)  [unwired: 6 in]
  n68 = Select(t=TRUE, s=w92, f=FALSE) -> (s? t:f=w47:bool)
  n69 = Select(t=TRUE, s=w90, f=FALSE) -> (s? t:f=w45:bool)
  n70 = Select(t=TRUE, s=w91, f=FALSE) -> (s? t:f=w46:bool)
  n71 = Select(t=TRUE, s=w115, f=FALSE) -> (s? t:f=w49:bool)
  n72 = Select(t=TRUE, s=w87, f=FALSE) -> (s? t:f=w42:bool)
  n73 = Select(t=TRUE, s=w93, f=FALSE) -> (s? t:f=w48:bool)
  n74 = Unbundle By Name("main ref") -> ("Config Parameters.SAMPLES"=w356:refnum<vi>)
  n75 = Unbundle By Name("main ref") -> ("Config Parameters.Heave Loop Delay"=w244:refnum<vi>)
  n76 = Unbundle By Name("main ref") -> ("Config Parameters.Heave PID Speed"=w245:refnum<vi>)
  n77 = Unbundle By Name("main ref") -> ("Config Parameters.Surge Jog Speed"=w249:refnum<vi>)
  n78 = Unbundle By Name("main ref") -> ("Config Parameters.Heave Jog Speed"=w250:refnum<vi>)
  n79 = Unbundle By Name("main ref") -> ("About Screen.Humidity Port:"=w350:refnum<vi>)
  n80 = Unbundle By Name("main ref") -> ("About Screen.Temp Modbus:"=w345:refnum<vi>)
  n81 = Unbundle By Name("main ref") -> ("About Screen.Heave and Surge COM Port:"=w344:refnum<vi>)
  n82 = Unbundle By Name("main ref") -> ("About Screen.Sway COM Port:"=w340:refnum<vi>)
  n83 = Unbundle By Name("main ref") -> ("About Screen.Ramp Port:"=w339:refnum<vi>)
  n84 = Unbundle By Name("main ref") -> ("About Screen.ECR Port:"=w336:refnum<vi>)
  n85 = Unbundle By Name("main ref") -> ("Config Parameters.Sway PPR"=w417:refnum<vi>)
  n86 = Unbundle By Name("main ref") -> ("Config Parameters.Sway Pitch"=w412:refnum<vi>)
  n87 = Unbundle By Name("main ref") -> ("Config Parameters.Surge PPR"=w406:refnum<vi>)
  n88 = Unbundle By Name("main ref") -> ("Config Parameters.Surge Pitch"=w411:refnum<vi>)
  n89 = Unbundle By Name("main ref") -> ("Config Parameters.Heave PPR"=w405:refnum<vi>)
  n90 = Unbundle By Name("main ref") -> ("Config Parameters.Heave Pitch"=w401:refnum<vi>)
  n91 = Unbundle By Name("main ref") -> ("Config Parameters.Heave distance"=w395:refnum<vi>)
  n92 = Unbundle By Name("main ref") -> ("Config Parameters.Surge distance (mm)"=w399:refnum<vi>)
  n93 = Unbundle By Name("main ref") -> ("Config Parameters.Sway distance (mm)"=w393:refnum<vi>)
  n94 = Unbundle By Name("main ref") -> ("Config Parameters.DataSavingLoopDelay(ms)"=w390:refnum<vi>)
  n95 = Unbundle By Name("main ref") -> ("Config Parameters.Acoustic Emission:"=w387:refnum<vi>)
  n96 = Unbundle By Name("main ref") -> ("Config Parameters.RotHomeSurgeOffsetCounts"=w384:refnum<vi>)
  n97 = Unbundle By Name("main ref") -> ("Config Parameters.RotHomeSwayOffsetCounts"=w381:refnum<vi>)
  n98 = Unbundle By Name("main ref") -> ("Config Parameters.TracHomeSurgeOffsetCounts 20MM"=w378:refnum<vi>)
  n99 = Unbundle By Name("main ref") -> ("Config Parameters.TracHomeSwayOffsetCounts 20MM"=w375:refnum<vi>)
  n100 = Unbundle By Name("main ref") -> ("Config Parameters.TracHomeSurgeOffsetCounts 10MM"=w371:refnum<vi>)
  n101 = Unbundle By Name("main ref") -> ("Config Parameters.TracHomeSwayOffsetCounts 10MM"=w374:refnum<vi>)
  n102 = Unbundle By Name("main ref") -> ("Config Parameters.LRMHomeSurgeOffsetCounts"=w365:refnum<vi>)
  n103 = Unbundle By Name("main ref") -> ("Config Parameters.LRMHomeSwayOffsetCounts"=w362:refnum<vi>)
  n104 = Unbundle By Name("main ref") -> ("Config Parameters.Filter%"=w361:refnum<vi>)
  n105 = Unbundle By Name("main ref") -> ("Config Parameters.Filter% 2"=w357:refnum<vi>)
  n106 = Unbundle By Name("main ref") -> ("Config Parameters.LOAD TRIP  ENABLE"=w136:refnum<vi>)
  n107 = Unbundle By Name("main ref") -> ("Config Parameters.DEPTH TRIP VALUE"=w137:refnum<vi>)
  n108 = Unbundle By Name("main ref") -> ("Config Parameters.LOAD TRIP VALUE"=w141:refnum<vi>)
  n109 = Unbundle By Name("main ref") -> ("Config Parameters.DEPTH TRIP   ENABLE"=w142:refnum<vi>)
  n110 = Unbundle By Name("main ref") -> ("Config Parameters.CYCLIC FF TRIP VALUE"=w148:refnum<vi>)
  n111 = Unbundle By Name("main ref") -> ("Config Parameters.FF TRIP VALUE"=w149:refnum<vi>)
  n112 = Unbundle By Name("main ref") -> ("Config Parameters.CYCLIC CoF TRIP VALUE"=w154:refnum<vi>)
  n113 = Unbundle By Name("main ref") -> ("Config Parameters.CYCLIC FF TRIP  ENABLE"=w155:refnum<vi>)
  n114 = Unbundle By Name("main ref") -> ("Config Parameters.FF TRIP  ENABLE"=w163:refnum<vi>)
  n115 = Unbundle By Name("main ref") -> ("Config Parameters.COF TRIP  ENABLE"=w158:refnum<vi>)
  n116 = Unbundle By Name("main ref") -> ("Config Parameters.JOG TRIP LOAD VALUE (N)"=w7:refnum<vi>)
  n117 = Unbundle By Name("main ref") -> ("Config Parameters.CYCLIC COF TRIP  ENABLE"=w131:refnum<vi>)
  n118 = Unbundle By Name("main ref") -> ("Config Parameters.COF TRIP VALUE"=w130:refnum<vi>)
  n119 = Unbundle By Name("main ref") -> ("Config Parameters.Sway Loop Delay"=w178:refnum<vi>)
  n120 = Unbundle By Name("main ref") -> ("Config Parameters.Sway PID Speed"=w174:refnum<vi>)
  n121 = Unbundle By Name("main ref") -> ("Config Parameters.Sway Jog Speed"=w173:refnum<vi>)
  n122 = property class="VISAName"(reference=w350, "Value"=w331) -> (reference out=w348:refnum<vi>, error out=w349:errorcluster)  [unwired: 1 in]
  n123 = property class="VISAName"(reference=w345, "Value"=w330) -> (reference out=w347:refnum<vi>, error out=w346:errorcluster)  [unwired: 1 in]
  n124 = Fract/Exp String To Number(string=w324) -> (number=w302:dbl)  [unwired: 3 in, 1 out]
  n125 = Fract/Exp String To Number(string=w323) -> (number=w301:dbl)  [unwired: 3 in, 1 out]
  n126 = Fract/Exp String To Number(string=w322) -> (number=w300:dbl)  [unwired: 3 in, 1 out]
  n127 = Fract/Exp String To Number(string=w321) -> (number=w299:dbl)  [unwired: 3 in, 1 out]
  n128 = Fract/Exp String To Number(string=w320) -> (number=w298:dbl)  [unwired: 3 in, 1 out]
  n129 = Fract/Exp String To Number(string=w319) -> (number=w297:dbl)  [unwired: 3 in, 1 out]
  n130 = Fract/Exp String To Number(string=w318) -> (number=w296:dbl)  [unwired: 3 in, 1 out]
  n131 = Fract/Exp String To Number(string=w317) -> (number=w295:dbl)  [unwired: 3 in, 1 out]
  n132 = Fract/Exp String To Number(string=w316) -> (number=w294:dbl)  [unwired: 3 in, 1 out]
  n133 = Fract/Exp String To Number(string=w315) -> (number=w293:dbl)  [unwired: 3 in, 1 out]
  n134 = Fract/Exp String To Number(string=w314) -> (number=w292:dbl)  [unwired: 3 in, 1 out]
  n135 = Fract/Exp String To Number(string=w313) -> (number=w291:dbl)  [unwired: 3 in, 1 out]
  n136 = Fract/Exp String To Number(string=w312) -> (number=w290:dbl)  [unwired: 3 in, 1 out]
  n137 = Fract/Exp String To Number(string=w311) -> (number=w289:dbl)  [unwired: 3 in, 1 out]
  n138 = Fract/Exp String To Number(string=w310) -> (number=w288:dbl)  [unwired: 3 in, 1 out]
  n139 = Fract/Exp String To Number(string=w309) -> (number=w287:dbl)  [unwired: 3 in, 1 out]
  n140 = Fract/Exp String To Number(string=w308) -> (number=w286:dbl)  [unwired: 3 in, 1 out]
  n141 = Fract/Exp String To Number(string=w307) -> (number=w285:dbl)  [unwired: 3 in, 1 out]
  n142 = Fract/Exp String To Number(string=w306) -> (number=w284:dbl)  [unwired: 3 in, 1 out]
  n143 = Fract/Exp String To Number(string=w305) -> (number=w283:dbl)  [unwired: 3 in, 1 out]
  n144 = Fract/Exp String To Number(string=w304) -> (number=w282:dbl)  [unwired: 3 in, 1 out]
  n145 = Fract/Exp String To Number(string=w303) -> (number=w281:dbl)  [unwired: 3 in, 1 out]
  n146 = Fract/Exp String To Number(string=w241) -> (number=w254:dbl)  [unwired: 3 in, 1 out]
  n147 = Fract/Exp String To Number(string=w240) -> (number=w255:dbl)  [unwired: 3 in, 1 out]
  n148 = Fract/Exp String To Number(string=w239) -> (number=w256:dbl)  [unwired: 3 in, 1 out]
  n149 = Fract/Exp String To Number(string=w238) -> (number=w257:dbl)  [unwired: 3 in, 1 out]
  n150 = Fract/Exp String To Number(string=w2) -> (number=w4:dbl)  [unwired: 3 in, 1 out]
  n151 = Fract/Exp String To Number(string=w50) -> (number=w37:dbl)  [unwired: 3 in, 1 out]
  n152 = Fract/Exp String To Number(string=w114) -> (number=w41:dbl)  [unwired: 3 in, 1 out]
  n153 = Fract/Exp String To Number(string=w111) -> (number=w43:dbl)  [unwired: 3 in, 1 out]
  n154 = Fract/Exp String To Number(string=w113) -> (number=w33:dbl)  [unwired: 3 in, 1 out]
  n155 = Fract/Exp String To Number(string=w109) -> (number=w44:dbl)  [unwired: 3 in, 1 out]
  n156 = Fract/Exp String To Number(string=w166) -> (number=w169:dbl)  [unwired: 3 in, 1 out]
  n157 = Fract/Exp String To Number(string=w165) -> (number=w168:dbl)  [unwired: 3 in, 1 out]
  n158 = Fract/Exp String To Number(string=w164) -> (number=w167:dbl)  [unwired: 3 in, 1 out]
  n159 = property class="VISAName"(reference=w344, "Value"=w329) -> (reference out=w342:refnum<vi>, error out=w343:errorcluster)  [unwired: 1 in]
  n160 = property class="VISAName"(reference=w340, "Value"=w328) -> (reference out=w335:refnum<vi>, error out=w341:errorcluster)  [unwired: 1 in]
  n161 = property class="VISAName"(reference=w339, "Value"=w327) -> (reference out=w334:refnum<vi>, error out=w338:errorcluster)  [unwired: 1 in]
  n162 = property class="VISAName"(reference=w336, "Value"=w326) -> (reference out=w333:refnum<vi>, error out=w337:errorcluster)  [unwired: 1 in]
  n163 = Fract/Exp String To Number(string=w110) -> (number=w29:dbl)  [unwired: 3 in, 1 out]
  n164 = property class="DigNum (strict)"(reference=w365, "Value"=w285) -> (reference out=w366:refnum<vi>, error out=w364:errorcluster)  [unwired: 1 in]
  n165 = property class="DigNum (strict)"(reference=w362, "Value"=w284) -> (reference out=w367:refnum<vi>, error out=w363:errorcluster)  [unwired: 1 in]
  n166 = property class="DigNum (strict)"(reference=w361, "Value"=w283) -> (reference out=w359:refnum<vi>, error out=w360:errorcluster)  [unwired: 1 in]
  n167 = property class="DigNum (strict)"(reference=w356, "Value"=w281) -> (reference out=w354:refnum<vi>, error out=w355:errorcluster)  [unwired: 1 in]
  n168 = property class="DigNum (strict)"(reference=w244, "Value"=w254) -> (reference out=w242:refnum<vi>, error out=w243:errorcluster)  [unwired: 1 in]
  n169 = property class="DigNum (strict)"(reference=w357, "Value"=w282) -> (reference out=w353:refnum<vi>, error out=w358:errorcluster)  [unwired: 1 in]
  n170 = property class="DigNum (strict)"(reference=w245, "Value"=w255) -> (reference out=w247:refnum<vi>, error out=w246:errorcluster)  [unwired: 1 in]
  n171 = property class="DigNum (strict)"(reference=w250, "Value"=w257) -> (reference out=w252:refnum<vi>, error out=w251:errorcluster)  [unwired: 1 in]
  n172 = property class="DigNum (strict)"(reference=w7, "Value"=w4) -> (reference out=w5:refnum<vi>, error out=w6:errorcluster)  [unwired: 1 in]
  n173 = property class="DigNum (strict)"(reference=w381, "Value"=w290) -> (reference out=w380:refnum<vi>, error out=w382:errorcluster)  [unwired: 1 in]
  n174 = property class="DigNum (strict)"(reference=w371, "Value"=w287) -> (reference out=w369:refnum<vi>, error out=w372:errorcluster)  [unwired: 1 in]
  n175 = property class="DigNum (strict)"(reference=w374, "Value"=w286) -> (reference out=w368:refnum<vi>, error out=w373:errorcluster)  [unwired: 1 in]
  n176 = property class="DigNum (strict)"(reference=w249, "Value"=w256) -> (reference out=w253:refnum<vi>, error out=w248:errorcluster)  [unwired: 1 in]
  n177 = property class="DigNum (strict)"(reference=w417, "Value"=w302) -> (reference out=w415:refnum<vi>, error out=w416:errorcluster)  [unwired: 1 in]
  n178 = property class="DigNum (strict)"(reference=w395, "Value"=w296) -> (reference out=w352:refnum<vi>, error out=w396:errorcluster)  [unwired: 1 in]
  n179 = property class="DigNum (strict)"(reference=w378, "Value"=w289) -> (reference out=w379:refnum<vi>, error out=w377:errorcluster)  [unwired: 1 in]
  n180 = property class="DigNum (strict)"(reference=w375, "Value"=w288) -> (reference out=w370:refnum<vi>, error out=w376:errorcluster)  [unwired: 1 in]
  n181 = property class="DigNum (strict)"(reference=w412, "Value"=w301) -> (reference out=w414:refnum<vi>, error out=w413:errorcluster)  [unwired: 1 in]
  n182 = property class="DigNum (strict)"(reference=w406, "Value"=w300) -> (reference out=w408:refnum<vi>, error out=w407:errorcluster)  [unwired: 1 in]
  n183 = property class="DigNum (strict)"(reference=w405, "Value"=w298) -> (reference out=w400:refnum<vi>, error out=w404:errorcluster)  [unwired: 1 in]
  n184 = property class="DigNum (strict)"(reference=w399, "Value"=w295) -> (reference out=w397:refnum<vi>, error out=w398:errorcluster)  [unwired: 1 in]
  n185 = property class="DigNum (strict)"(reference=w393, "Value"=w294) -> (reference out=w392:refnum<vi>, error out=w394:errorcluster)  [unwired: 1 in]
  n186 = property class="DigNum (strict)"(reference=w390, "Value"=w293) -> (reference out=w391:refnum<vi>, error out=w389:errorcluster)  [unwired: 1 in]
  n187 = property class="DigNum (strict)"(reference=w387, "Value"=w292) -> (reference out=w386:refnum<vi>, error out=w388:errorcluster)  [unwired: 1 in]
  n188 = property class="DigNum (strict)"(reference=w384, "Value"=w291) -> (reference out=w385:refnum<vi>, error out=w383:errorcluster)  [unwired: 1 in]
  n189 = property class="DigNum (strict)"(reference=w411, "Value"=w299) -> (reference out=w409:refnum<vi>, error out=w410:errorcluster)  [unwired: 1 in]
  n190 = property class="DigNum (strict)"(reference=w401, "Value"=w297) -> (reference out=w403:refnum<vi>, error out=w402:errorcluster)  [unwired: 1 in]
  n191 = property class="DigNum (strict)"(reference=w178, "Value"=w169) -> (reference out=w176:refnum<vi>, error out=w177:errorcluster)  [unwired: 1 in]
  n192 = property class="DigNum (strict)"(reference=w173, "Value"=w167) -> (reference out=w171:refnum<vi>, error out=w172:errorcluster)  [unwired: 1 in]
  n193 = property class="DigNum (strict)"(reference=w137, "Value"=w41) -> (reference out=w139:refnum<vi>, error out=w138:errorcluster)  [unwired: 1 in]
  n194 = property class="DigNum (strict)"(reference=w148, "Value"=w43) -> (reference out=w146:refnum<vi>, error out=w147:errorcluster)  [unwired: 1 in]
  n195 = property class="DigNum (strict)"(reference=w149, "Value"=w29) -> (reference out=w151:refnum<vi>, error out=w150:errorcluster)  [unwired: 1 in]
  n196 = property class="DigNum (strict)"(reference=w154, "Value"=w44) -> (reference out=w152:refnum<vi>, error out=w153:errorcluster)  [unwired: 1 in]
  n197 = property class="DigNum (strict)"(reference=w174, "Value"=w168) -> (reference out=w170:refnum<vi>, error out=w175:errorcluster)  [unwired: 1 in]
  n198 = property class="DigNum (strict)"(reference=w141, "Value"=w33) -> (reference out=w145:refnum<vi>, error out=w140:errorcluster)  [unwired: 1 in]
  n199 = property class="Bool (strict)"(reference=w131, "Value"=w49) -> (reference out=w133:refnum<vi>, error out=w132:errorcluster)  [unwired: 1 in]
  n200 = property class="DigNum (strict)"(reference=w130, "Value"=w37) -> (reference out=w128:refnum<vi>, error out=w129:errorcluster)  [unwired: 1 in]
  n201 = property class="Bool (strict)"(reference=w142, "Value"=w42) -> (reference out=w144:refnum<vi>, error out=w143:errorcluster)  [unwired: 1 in]
  n202 = property class="Bool (strict)"(reference=w155, "Value"=w45) -> (reference out=w157:refnum<vi>, error out=w156:errorcluster)  [unwired: 1 in]
  n203 = property class="Bool (strict)"(reference=w163, "Value"=w46) -> (reference out=w161:refnum<vi>, error out=w162:errorcluster)  [unwired: 1 in]
  n204 = property class="Bool (strict)"(reference=w158, "Value"=w47) -> (reference out=w160:refnum<vi>, error out=w159:errorcluster)  [unwired: 1 in]
  n205 = property class="Bool (strict)"(reference=w136, "Value"=w48) -> (reference out=w134:refnum<vi>, error out=w135:errorcluster)  [unwired: 1 in]
  n206 = Close Reference(reference=w348, error in (no error)=w349) -> ()  [unwired: 1 out]
  n207 = Close Reference(reference=w347, error in (no error)=w346) -> ()  [unwired: 1 out]
  n208 = Close Reference(reference=w342, error in (no error)=w343) -> ()  [unwired: 1 out]
  n209 = Close Reference(reference=w335, error in (no error)=w341) -> ()  [unwired: 1 out]
  n210 = Close Reference(reference=w334, error in (no error)=w338) -> ()  [unwired: 1 out]
  n211 = Close Reference(reference=w333, error in (no error)=w337) -> ()  [unwired: 1 out]
  n212 = Close Reference(reference=w366, error in (no error)=w364) -> ()  [unwired: 1 out]
  n213 = Close Reference(reference=w367, error in (no error)=w363) -> ()  [unwired: 1 out]
  n214 = Close Reference(reference=w359, error in (no error)=w360) -> ()  [unwired: 1 out]
  n215 = Close Reference(reference=w354, error in (no error)=w355) -> ()  [unwired: 1 out]
  n216 = Close Reference(reference=w242, error in (no error)=w243) -> ()  [unwired: 1 out]
  n217 = Close Reference(reference=w353, error in (no error)=w358) -> ()  [unwired: 1 out]
  n218 = Close Reference(reference=w247, error in (no error)=w246) -> ()  [unwired: 1 out]
  n219 = Close Reference(reference=w252, error in (no error)=w251) -> ()  [unwired: 1 out]
  n220 = Close Reference(reference=w5, error in (no error)=w6) -> ()  [unwired: 1 out]
  n221 = Close Reference(reference=w380, error in (no error)=w382) -> ()  [unwired: 1 out]
  n222 = Close Reference(reference=w369, error in (no error)=w372) -> ()  [unwired: 1 out]
  n223 = Close Reference(reference=w368, error in (no error)=w373) -> ()  [unwired: 1 out]
  n224 = Close Reference(reference=w253, error in (no error)=w248) -> ()  [unwired: 1 out]
  n225 = Close Reference(reference=w415, error in (no error)=w416) -> ()  [unwired: 1 out]
  n226 = Close Reference(reference=w352, error in (no error)=w396) -> ()  [unwired: 1 out]
  n227 = Close Reference(reference=w379, error in (no error)=w377) -> ()  [unwired: 1 out]
  n228 = Close Reference(reference=w370, error in (no error)=w376) -> ()  [unwired: 1 out]
  n229 = Close Reference(reference=w414, error in (no error)=w413) -> ()  [unwired: 1 out]
  n230 = Close Reference(reference=w408, error in (no error)=w407) -> ()  [unwired: 1 out]
  n231 = Close Reference(reference=w400, error in (no error)=w404) -> ()  [unwired: 1 out]
  n232 = Close Reference(reference=w397, error in (no error)=w398) -> ()  [unwired: 1 out]
  n233 = Close Reference(reference=w392, error in (no error)=w394) -> ()  [unwired: 1 out]
  n234 = Close Reference(reference=w391, error in (no error)=w389) -> ()  [unwired: 1 out]
  n235 = Close Reference(reference=w386, error in (no error)=w388) -> ()  [unwired: 1 out]
  n236 = Close Reference(reference=w385, error in (no error)=w383) -> ()  [unwired: 1 out]
  n237 = Close Reference(reference=w409, error in (no error)=w410) -> ()  [unwired: 1 out]
  n238 = Close Reference(reference=w403, error in (no error)=w402) -> ()  [unwired: 1 out]
  n239 = Close Reference(reference=w133, error in (no error)=w132) -> ()  [unwired: 1 out]
  n240 = Close Reference(reference=w176, error in (no error)=w177) -> ()  [unwired: 1 out]
  n241 = Close Reference(reference=w171, error in (no error)=w172) -> ()  [unwired: 1 out]
  n242 = Close Reference(reference=w139, error in (no error)=w138) -> ()  [unwired: 1 out]
  n243 = Close Reference(reference=w144, error in (no error)=w143) -> ()  [unwired: 1 out]
  n244 = Close Reference(reference=w146, error in (no error)=w147) -> ()  [unwired: 1 out]
  n245 = Close Reference(reference=w151, error in (no error)=w150) -> ()  [unwired: 1 out]
  n246 = Close Reference(reference=w152, error in (no error)=w153) -> ()  [unwired: 1 out]
  n247 = Close Reference(reference=w157, error in (no error)=w156) -> ()  [unwired: 1 out]
  n248 = Close Reference(reference=w161, error in (no error)=w162) -> ()  [unwired: 1 out]
  n249 = Close Reference(reference=w160, error in (no error)=w159) -> ()  [unwired: 1 out]
  n250 = Close Reference(reference=w134, error in (no error)=w135) -> ()  [unwired: 1 out]
  n251 = Close Reference(reference=w170, error in (no error)=w175) -> ()  [unwired: 1 out]
  n252 = Close Reference(reference=w145, error in (no error)=w140) -> ()  [unwired: 1 out]
  n253 = Close Reference(reference=w128, error in (no error)=w129) -> ()  [unwired: 1 out]
  n254 = for {
    tunnel: "NEW PID PARAMETERS" ("WRITE /READ SECTION") -> [w492]
    tunnel: [w491] -> w235
    tunnel: string[] ["PID DELAY (sec)", "Kp", "Ki", "Kd", "Deaadband", "pct_scale", "Init_step", "i_limit", "Max Step Limit", "Min_pos_limit", "Max_pos_limit", "Fine_tune_zone", "min_deadband_floor", "min_finetune_floor", "dynamic_spindle_noise_scalar", "filter_alpha"] -> [w488] mode=indexing
    tunnel: [w487] -> w208 mode=indexing
    tunnel: w236 -> [w486]
    n255 = call "CONFIG FILE MAIN Unitest.vi"("WRITE /READ SECTION"=w492, "READ KEY"=w488, "error in"=w486, "PARAMETER/CONFIG"=TRUE, "Config Enum"=Config_file__FGV_Unitest_enum."READ") -> ("READ VALUE"=w487:string, "error out"=w491:errorcluster)  [unwired: 13 in]
  }
  n256 = Unbundle By Name("main ref") -> ("Loading.Enter the CoF Trip"=w40:refnum<vi>)
  n257 = Unbundle By Name("main ref") -> ("Main Screen.Load Disable Trip"=w78:refnum<vi>)
  n258 = Unbundle By Name("main ref") -> ("Main Screen.FF Disable Trip"=w51:refnum<vi>)
  n259 = Unbundle By Name("main ref") -> ("Main Screen.COF Disable Trip"=w56:refnum<vi>)
  n260 = Unbundle By Name("main ref") -> ("Main Screen.Cyclic FF Disable Trip"=w59:refnum<vi>)
  n261 = Unbundle By Name("main ref") -> ("Main Screen.cyclic COF Disable Trip"=w83:refnum<vi>)
  n262 = Unbundle By Name("main ref") -> ("Main Screen.FF TRIP"=w65:refnum<vi>)
  n263 = Unbundle By Name("main ref") -> ("Main Screen.COF TRIP"=w84:refnum<vi>)
  n264 = Unbundle By Name("main ref") -> ("Main Screen.Depth Trip"=w77:refnum<vi>)
  n265 = Unbundle By Name("main ref") -> ("Main Screen.Depth Trip 2"=w72:refnum<vi>)
  n266 = Unbundle By Name("main ref") -> ("Main Screen.Cyclic FF TRIP"=w66:refnum<vi>)
  n267 = Unbundle By Name("main ref") -> ("Main Screen.cyclic COF TRIP"=w60:refnum<vi>)
  n268 = Unbundle By Name("main ref") -> ("Main Screen.NL Trip 2"=w73:refnum<vi>)
  n269 = Unbundle By Name("main ref") -> ("New PID LOGIC.PID SDelay"=w232:refnum<vi>)
  n270 = Unbundle By Name("main ref") -> ("New PID LOGIC.Kp"=w231:refnum<vi>)
  n271 = Unbundle By Name("main ref") -> ("New PID LOGIC.Ki"=w226:refnum<vi>)
  n272 = Unbundle By Name("main ref") -> ("New PID LOGIC.Kd"=w225:refnum<vi>)
  n273 = Unbundle By Name("main ref") -> ("New PID LOGIC.Deadband"=w221:refnum<vi>)
  n274 = Unbundle By Name("main ref") -> ("New PID LOGIC.pct_scale"=w220:refnum<vi>)
  n275 = Unbundle By Name("main ref") -> ("New PID LOGIC.Init Step"=w217:refnum<vi>)
  n276 = Unbundle By Name("main ref") -> ("New PID LOGIC.i_limit"=w216:refnum<vi>)
  n277 = Unbundle By Name("main ref") -> ("New PID LOGIC.Max Step Linit"=w213:refnum<vi>)
  n278 = Unbundle By Name("main ref") -> ("New PID LOGIC.Max_pos_limit"=w211:refnum<vi>)
  n279 = Unbundle By Name("main ref") -> ("New PID LOGIC.Min_pos_limit"=w210:refnum<vi>)
  n280 = Unbundle By Name("main ref") -> ("New PID LOGIC.min_deadband_floor"=w28:refnum<vi>)
  n281 = Unbundle By Name("main ref") -> ("New PID LOGIC.min_finetune_floor"=w25:refnum<vi>)
  n282 = Unbundle By Name("main ref") -> ("New PID LOGIC.dynamic_spindle_noise_scalar"=w23:refnum<vi>)
  n283 = Unbundle By Name("main ref") -> ("New PID LOGIC.filter_alpha"=w22:refnum<vi>)
  n284 = Index Array(array=w208) -> (element #1=w207:string, element #2=w206:string, element #3=w203:string, element #4=w202:string, element #5=w201:string, element #6=w200:string, element #7=w195:string, element #8=w194:string, element #9=w193:string, element #10=w192:string, element #11=w191:string, element #12=w13:string, element #13=w12:string, element #14=w11:string, element #15=w10:string)  [unwired: 15 in]
  n285 = property class="DigNum (strict)"(reference=w40, "Value"=w37) -> (reference out=w38:refnum<vi>, error out=w39:errorcluster)  [unwired: 1 in]
  n286 = property class="DigNum (strict)"(reference=w77, "Value"=w41) -> (reference out=w75:refnum<vi>, error out=w76:errorcluster)  [unwired: 1 in]
  n287 = property class="DigNum (strict)"(reference=w66, "Value"=w43) -> (reference out=w68:refnum<vi>, error out=w67:errorcluster)  [unwired: 1 in]
  n288 = property class="DigNum (strict)"(reference=w65, "Value"=w29) -> (reference out=w63:refnum<vi>, error out=w64:errorcluster)  [unwired: 1 in]
  n289 = property class="DigNum (strict)"(reference=w60, "Value"=w44) -> (reference out=w62:refnum<vi>, error out=w61:errorcluster)  [unwired: 1 in]
  n290 = property class="DigNum (strict)"(reference=w73, "Value"=w33) -> (reference out=w69:refnum<vi>, error out=w74:errorcluster)  [unwired: 1 in]
  n291 = property class="Bool (strict)"(reference=w83, "Value"=w49) -> (reference out=w81:refnum<vi>, error out=w82:errorcluster)  [unwired: 1 in]
  n292 = property class="DigNum (strict)"(reference=w84, "Value"=w37) -> (reference out=w86:refnum<vi>, error out=w85:errorcluster)  [unwired: 1 in]
  n293 = property class="Bool (strict)"(reference=w72, "Value"=w42) -> (reference out=w70:refnum<vi>, error out=w71:errorcluster)  [unwired: 1 in]
  n294 = property class="Bool (strict)"(reference=w59, "Value"=w45) -> (reference out=w57:refnum<vi>, error out=w58:errorcluster)  [unwired: 1 in]
  n295 = property class="Bool (strict)"(reference=w51, "Value"=w46) -> (reference out=w53:refnum<vi>, error out=w52:errorcluster)  [unwired: 1 in]
  n296 = property class="Bool (strict)"(reference=w56, "Value"=w47) -> (reference out=w54:refnum<vi>, error out=w55:errorcluster)  [unwired: 1 in]
  n297 = property class="Bool (strict)"(reference=w78, "Value"=w48) -> (reference out=w80:refnum<vi>, error out=w79:errorcluster)  [unwired: 1 in]
  n298 = call "CONFIG FILE MAIN Unitest.vi"("error in"=w235, "Config Enum"=Config_file__FGV_Unitest_enum."CLOSE") -> ("error out"=→"error out":errorcluster)  [unwired: 16 in, 1 out]
  n299 = Unbundle By Name("main ref") -> ("Loading.Enter the Normal load Trip"=w36:refnum<vi>)
  n300 = Fract/Exp String To Number(string=w207) -> (number=w205:dbl)  [unwired: 3 in, 1 out]
  n301 = Fract/Exp String To Number(string=w206) -> (number=w204:dbl)  [unwired: 3 in, 1 out]
  n302 = Fract/Exp String To Number(string=w203) -> (number=w199:dbl)  [unwired: 3 in, 1 out]
  n303 = Fract/Exp String To Number(string=w13) -> (number=w20:dbl)  [unwired: 3 in, 1 out]
  n304 = Fract/Exp String To Number(string=w12) -> (number=w19:dbl)  [unwired: 3 in, 1 out]
  n305 = Fract/Exp String To Number(string=w11) -> (number=w18:dbl)  [unwired: 3 in, 1 out]
  n306 = Fract/Exp String To Number(string=w10) -> (number=w17:dbl)  [unwired: 3 in, 1 out]
  n307 = Close Reference(reference=w38, error in (no error)=w39) -> ()  [unwired: 1 out]
  n308 = Fract/Exp String To Number(string=w202) -> (number=w198:dbl)  [unwired: 3 in, 1 out]
  n309 = Fract/Exp String To Number(string=w201) -> (number=w197:dbl)  [unwired: 3 in, 1 out]
  n310 = Fract/Exp String To Number(string=w200) -> (number=w196:dbl)  [unwired: 3 in, 1 out]
  n311 = Fract/Exp String To Number(string=w195) -> (number=w190:dbl)  [unwired: 3 in, 1 out]
  n312 = Fract/Exp String To Number(string=w194) -> (number=w189:dbl)  [unwired: 3 in, 1 out]
  n313 = Fract/Exp String To Number(string=w193) -> (number=w188:dbl)  [unwired: 3 in, 1 out]
  n314 = Fract/Exp String To Number(string=w192) -> (number=w187:dbl)  [unwired: 3 in, 1 out]
  n315 = Fract/Exp String To Number(string=w191) -> (number=w186:dbl)  [unwired: 3 in, 1 out]
  n316 = Close Reference(reference=w81, error in (no error)=w82) -> ()  [unwired: 1 out]
  n317 = Unbundle By Name("main ref") -> ("Loading.Enter the Friction Force Trip"=w32:refnum<vi>)
  n318 = Close Reference(reference=w75, error in (no error)=w76) -> ()  [unwired: 1 out]
  n319 = Close Reference(reference=w70, error in (no error)=w71) -> ()  [unwired: 1 out]
  n320 = Close Reference(reference=w68, error in (no error)=w67) -> ()  [unwired: 1 out]
  n321 = Close Reference(reference=w63, error in (no error)=w64) -> ()  [unwired: 1 out]
  n322 = Close Reference(reference=w62, error in (no error)=w61) -> ()  [unwired: 1 out]
  n323 = Close Reference(reference=w57, error in (no error)=w58) -> ()  [unwired: 1 out]
  n324 = Close Reference(reference=w53, error in (no error)=w52) -> ()  [unwired: 1 out]
  n325 = Close Reference(reference=w54, error in (no error)=w55) -> ()  [unwired: 1 out]
  n326 = Close Reference(reference=w80, error in (no error)=w79) -> ()  [unwired: 1 out]
  n327 = Close Reference(reference=w69, error in (no error)=w74) -> ()  [unwired: 1 out]
  n328 = Close Reference(reference=w86, error in (no error)=w85) -> ()  [unwired: 1 out]
  n329 = property class="DigNum (strict)"(reference=w232, "Value"=w205) -> (reference out=w234:refnum<vi>, error out=w233:errorcluster)  [unwired: 1 in]
  n330 = property class="DigNum (strict)"(reference=w231, "Value"=w204) -> (reference out=w229:refnum<vi>, error out=w230:errorcluster)  [unwired: 1 in]
  n331 = property class="DigNum (strict)"(reference=w226, "Value"=w199) -> (reference out=w228:refnum<vi>, error out=w227:errorcluster)  [unwired: 1 in]
  n332 = property class="DigNum (strict)"(reference=w28, "Value"=w20) -> (reference out=w9:refnum<vi>, error out=w27:errorcluster)  [unwired: 1 in]
  n333 = property class="DigNum (strict)"(reference=w25, "Value"=w19) -> (reference out=w16:refnum<vi>, error out=w26:errorcluster)  [unwired: 1 in]
  n334 = property class="DigNum (strict)"(reference=w23, "Value"=w18) -> (reference out=w15:refnum<vi>, error out=w24:errorcluster)  [unwired: 1 in]
  n335 = property class="DigNum (strict)"(reference=w22, "Value"=w17) -> (reference out=w14:refnum<vi>, error out=w21:errorcluster)  [unwired: 1 in]
  n336 = property class="DigNum (strict)"(reference=w225, "Value"=w198) -> (reference out=w223:refnum<vi>, error out=w224:errorcluster)  [unwired: 1 in]
  n337 = property class="DigNum (strict)"(reference=w221, "Value"=w197) -> (reference out=w184:refnum<vi>, error out=w222:errorcluster)  [unwired: 1 in]
  n338 = property class="DigNum (strict)"(reference=w220, "Value"=w196) -> (reference out=w185:refnum<vi>, error out=w219:errorcluster)  [unwired: 1 in]
  n339 = property class="DigNum (strict)"(reference=w217, "Value"=w190) -> (reference out=w183:refnum<vi>, error out=w218:errorcluster)  [unwired: 1 in]
  n340 = property class="DigNum (strict)"(reference=w216, "Value"=w189) -> (reference out=w182:refnum<vi>, error out=w215:errorcluster)  [unwired: 1 in]
  n341 = property class="DigNum (strict)"(reference=w213, "Value"=w188) -> (reference out=w181:refnum<vi>, error out=w214:errorcluster)  [unwired: 1 in]
  n342 = property class="DigNum (strict)"(reference=w211, "Value"=w187) -> (reference out=w180:refnum<vi>, error out=w212:errorcluster)  [unwired: 1 in]
  n343 = property class="DigNum (strict)"(reference=w210, "Value"=w186) -> (reference out=w179:refnum<vi>, error out=w209:errorcluster)  [unwired: 1 in]
  n344 = property class="DigNum (strict)"(reference=w36, "Value"=w33) -> (reference out=w34:refnum<vi>, error out=w35:errorcluster)  [unwired: 1 in]
  n345 = property class="DigNum (strict)"(reference=w32, "Value"=w29) -> (reference out=w30:refnum<vi>, error out=w31:errorcluster)  [unwired: 1 in]
  n346 = Close Reference(reference=w234, error in (no error)=w233) -> ()  [unwired: 1 out]
  n347 = Close Reference(reference=w229, error in (no error)=w230) -> ()  [unwired: 1 out]
  n348 = Close Reference(reference=w228, error in (no error)=w227) -> ()  [unwired: 1 out]
  n349 = Close Reference(reference=w9, error in (no error)=w27) -> ()  [unwired: 1 out]
  n350 = Close Reference(reference=w16, error in (no error)=w26) -> ()  [unwired: 1 out]
  n351 = Close Reference(reference=w15, error in (no error)=w24) -> ()  [unwired: 1 out]
  n352 = Close Reference(reference=w14, error in (no error)=w21) -> ()  [unwired: 1 out]
  n353 = Close Reference(reference=w223, error in (no error)=w224) -> ()  [unwired: 1 out]
  n354 = Close Reference(reference=w184, error in (no error)=w222) -> ()  [unwired: 1 out]
  n355 = Close Reference(reference=w185, error in (no error)=w219) -> ()  [unwired: 1 out]
  n356 = Close Reference(reference=w183, error in (no error)=w218) -> ()  [unwired: 1 out]
  n357 = Close Reference(reference=w182, error in (no error)=w215) -> ()  [unwired: 1 out]
  n358 = Close Reference(reference=w181, error in (no error)=w214) -> ()  [unwired: 1 out]
  n359 = Close Reference(reference=w180, error in (no error)=w212) -> ()  [unwired: 1 out]
  n360 = Close Reference(reference=w179, error in (no error)=w209) -> ()  [unwired: 1 out]
  n361 = Close Reference(reference=w34, error in (no error)=w35) -> ()  [unwired: 1 out]
  n362 = Close Reference(reference=w30, error in (no error)=w31) -> ()  [unwired: 1 out]
